vi "Update VI Properties.vi"() -> ()   [LabVIEW 2016, in "update vi properties.lvlib"]
uses:
  update vi properties.lvlib
  support/user action.ctl
  support/Event Data.ctl
  support/Cluster_Data.ctl
  <vilib>/picture/picture.llb/imagedata.ctl
panel:
  in  "Adjust all Controls & Indicators":bool=TRUE
  in  "Prompt?":bool
  in  "Set all VIs":bool
  in  "Load":bool
  in  "Error in":errorcluster
  in  "Event Data":T1
  in  "Controls":string[][](table)
  in  "Indicators":string[][](table)
  in  "Help Tag":string
  in  "Help Path":string
  out "Path to VI":string
  in  "VI Description":string
  out "VI Conn Pane":picture
  in  "Select a VI to View/Edit Properties:":i32(listbox)=-1
  in  "Action":T2
  in  "OK":bool
  in  "Cancel":bool
  in  "Apply":bool
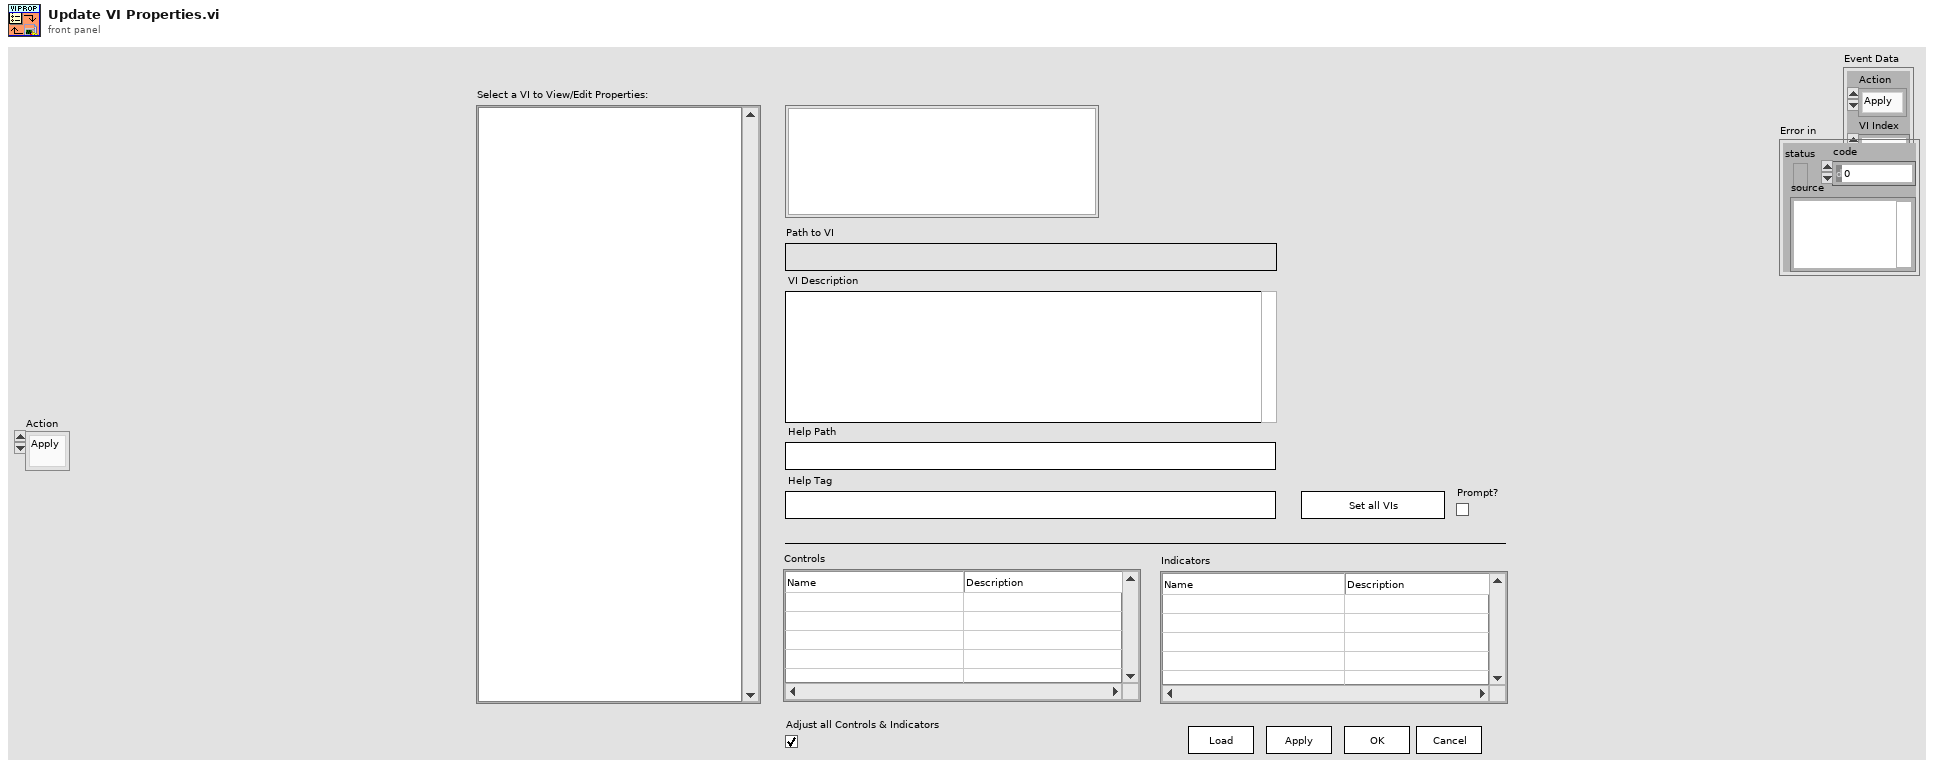
[diagram p1: front panel]
types:
  T1 = typedef "update vi properties.lvlib/Event Data.ctl" = cluster{"Action":T2, "VI Index":i32}
  T2 = typedef "update vi properties.lvlib/user action.ctl" = enum16{"Apply", "Cancel", "VI Selected", "Value Changed", "Set all VIs", "Controls/Indicator Changed", "Load VIs"}
  T3 = typedef "update vi properties.lvlib/Cluster_Data.ctl" = cluster{"changed?":bool, "VI Data":string[], "Controls":string[][], "Indicator":string[][], "Conpane Img":T4}
  T4 = typedef "imagedata.ctl" = cluster{"image type":i32, "image depth":i32, "image":u8[], "mask":u8[], "colors":u32[], "Rectangle":cluster{"left":i16, "top":i16, "right":i16, "bottom":i16}}
  T5 = enum32{"invalid VI type", "Standard VI", "Control VI", "Global VI", "Polymorphic VI", "Configuration VI", "SubSystem", "Facade VI", "Method VI", "Statechart Diagram VI"}
  T6 = enum8{"Enabled", "Disabled", "Disabled and Grayed Out"}
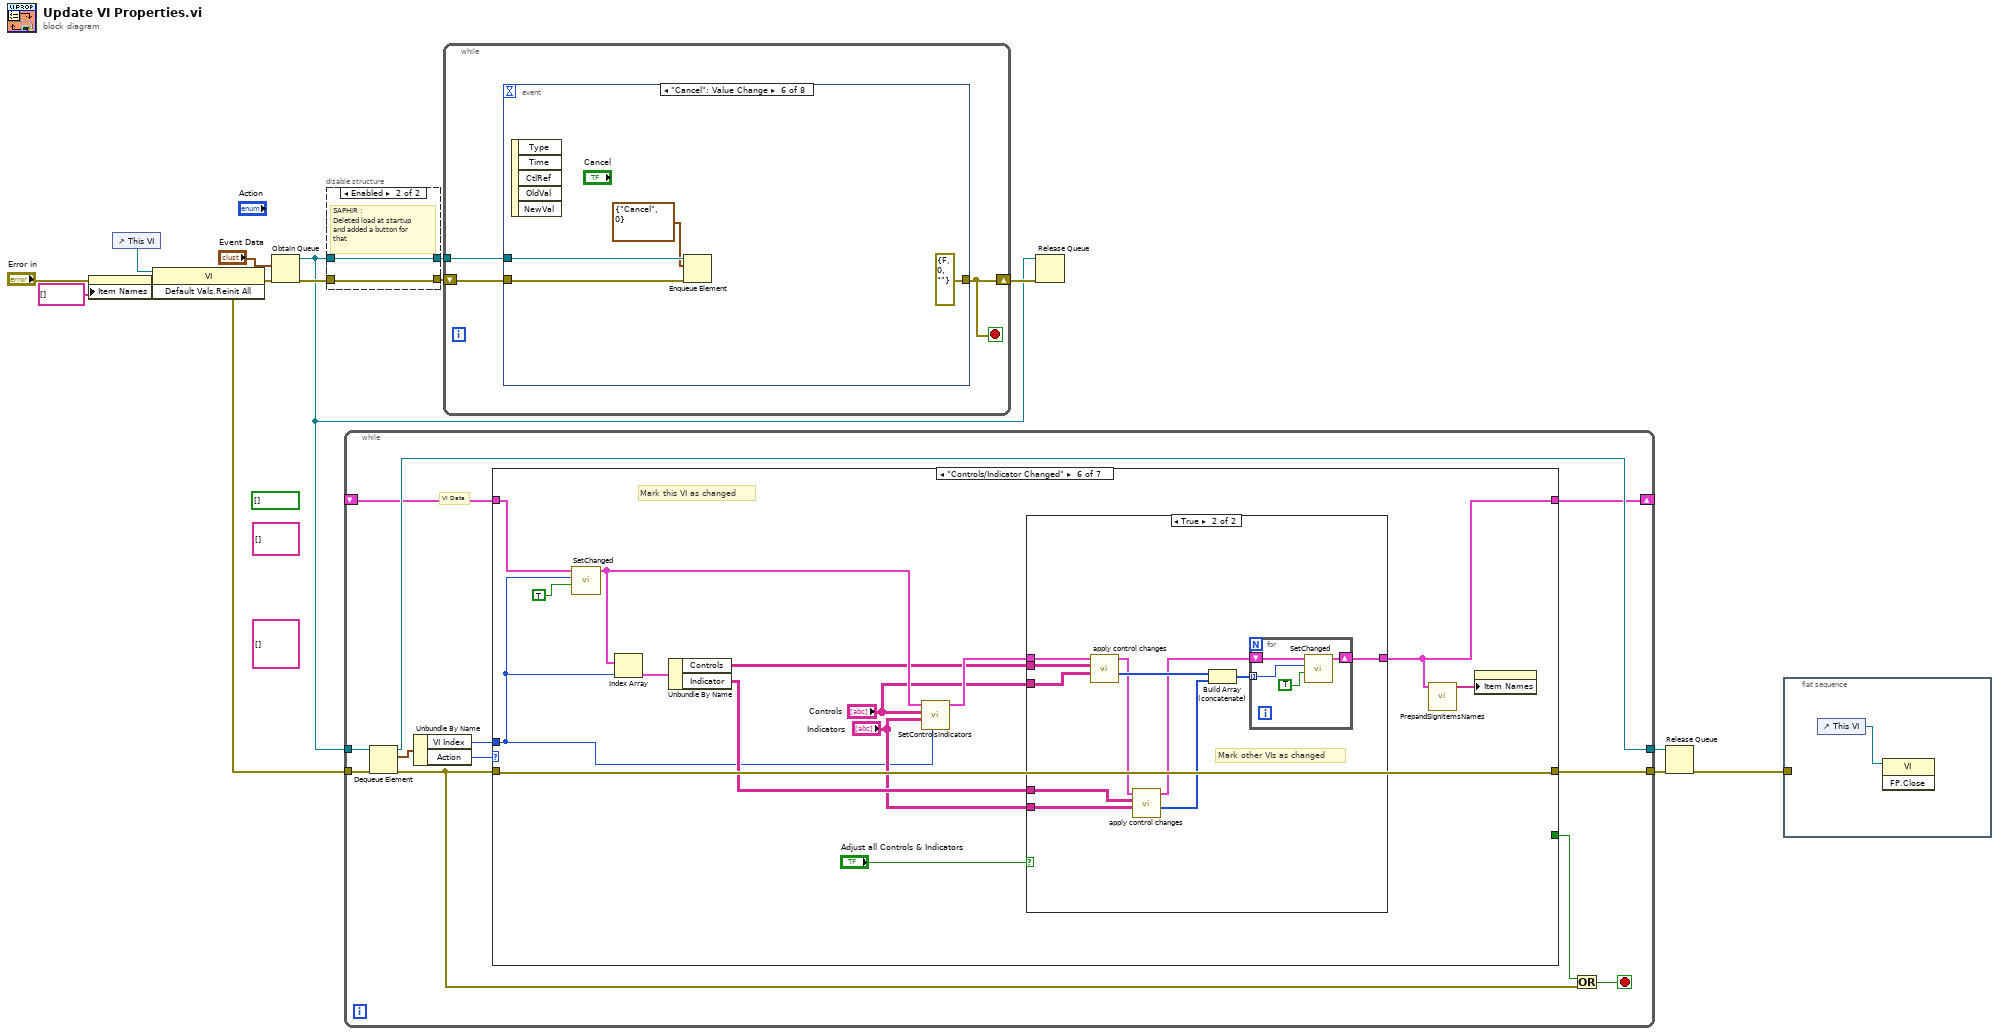
[diagram p0: block diagram]
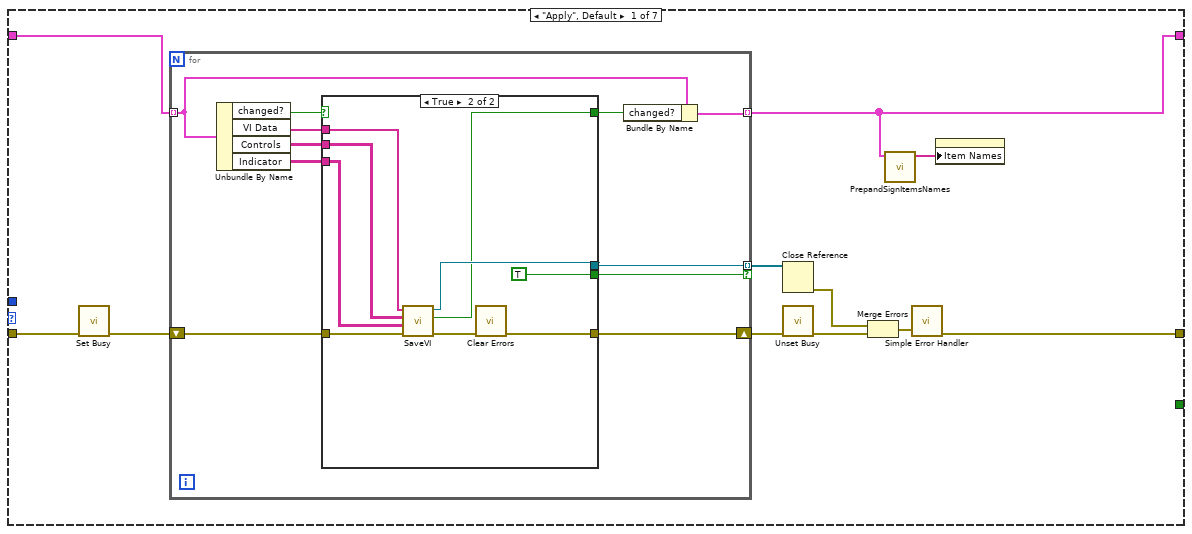
[diagram p2: hidden frame]
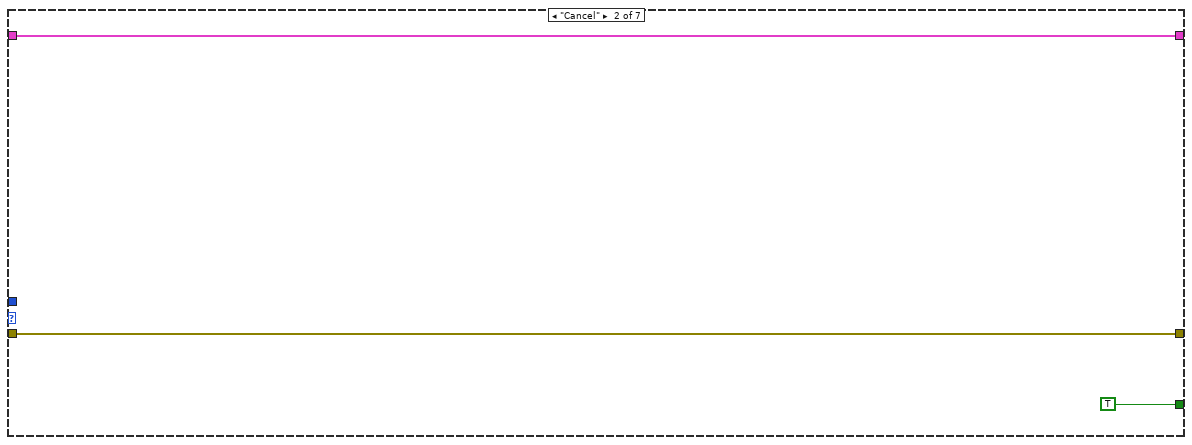
[diagram p4: hidden frame]
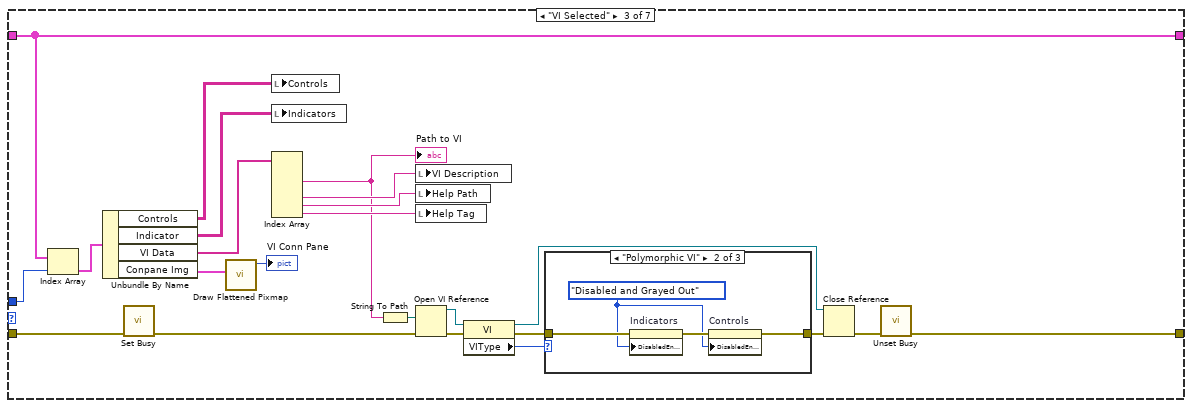
[diagram p5: hidden frame]
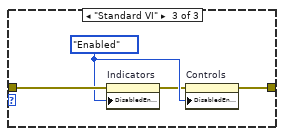
[diagram p7: hidden frame]
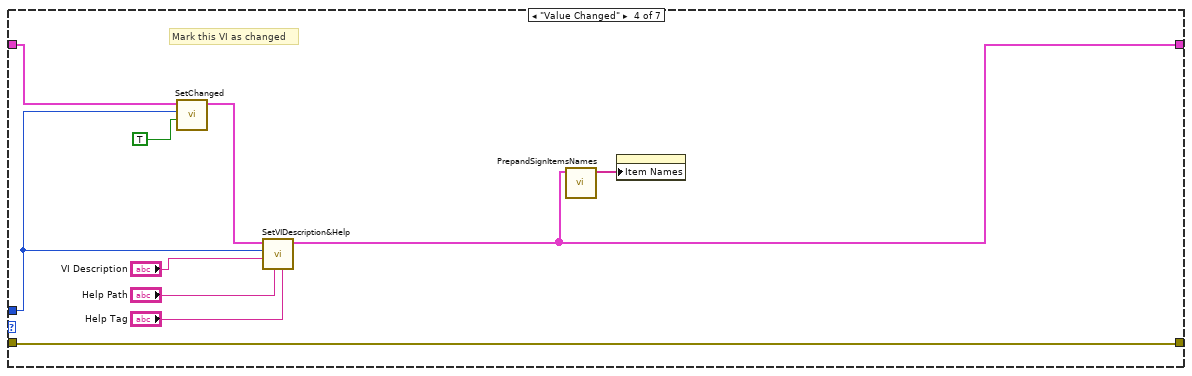
[diagram p8: hidden frame]
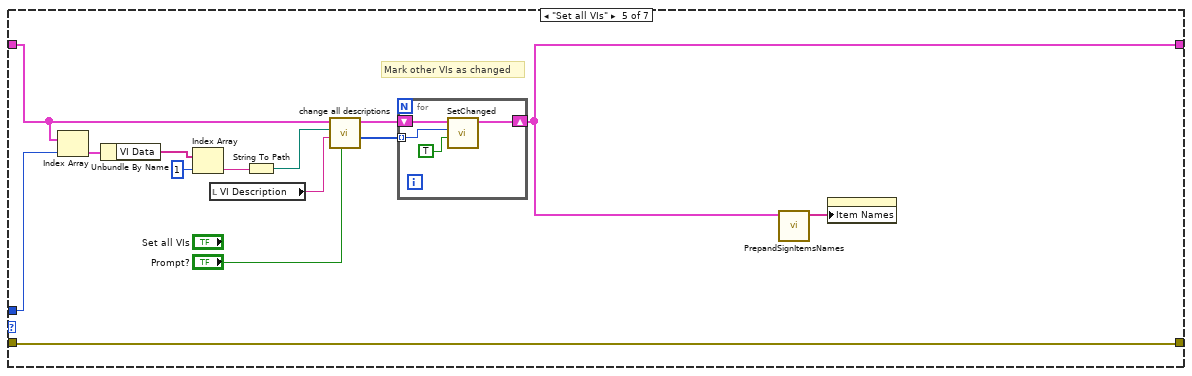
[diagram p9: hidden frame]
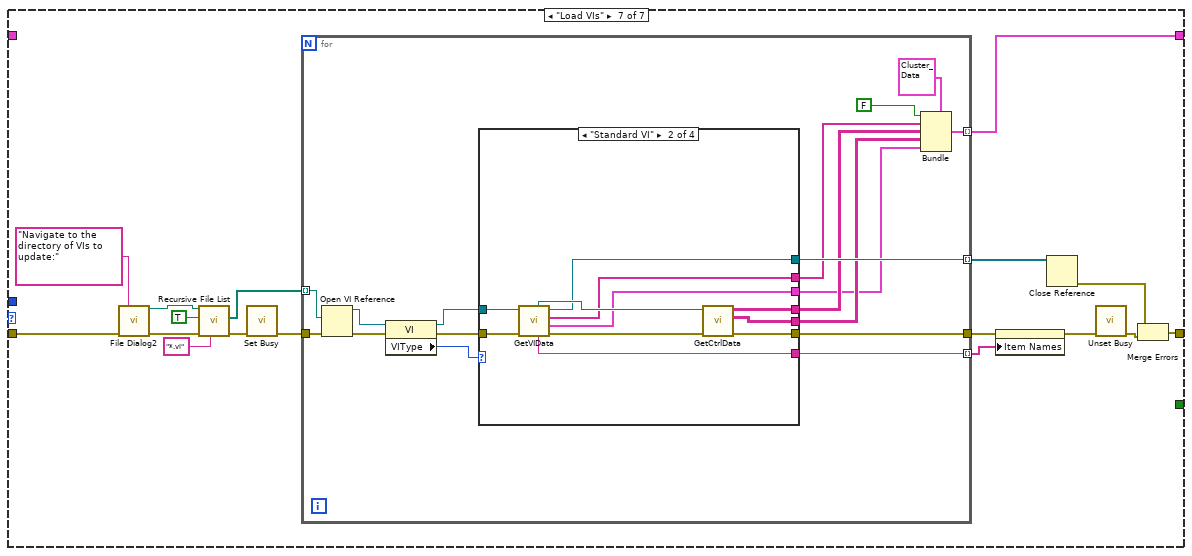
[diagram p11: hidden frame]
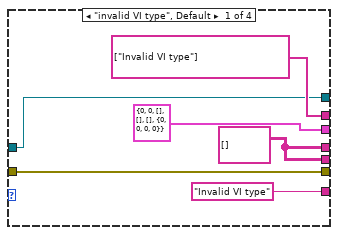
[diagram p12: hidden frame]
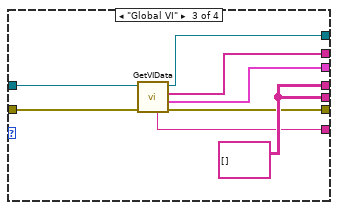
[diagram p13: hidden frame]
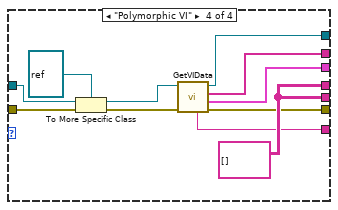
[diagram p14: hidden frame]
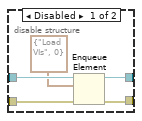
[diagram p15: hidden frame]
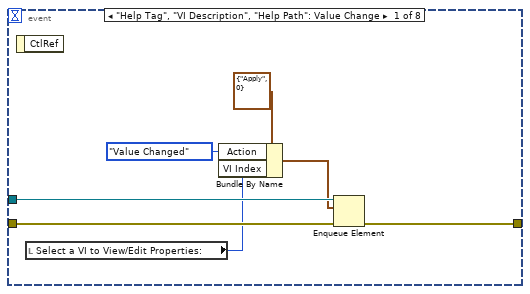
[diagram p16: hidden frame]
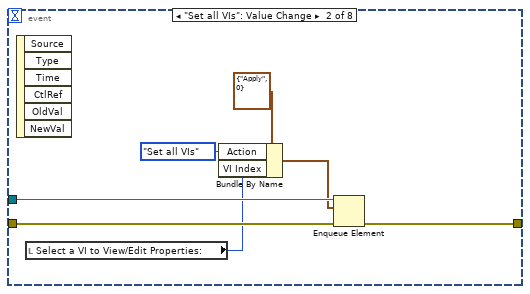
[diagram p17: hidden frame]
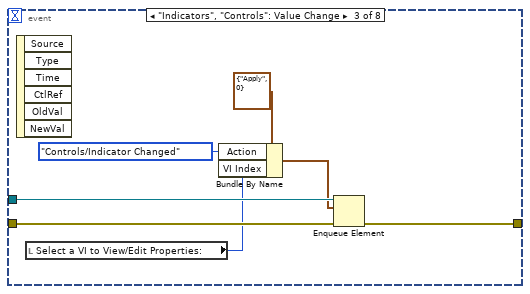
[diagram p18: hidden frame]
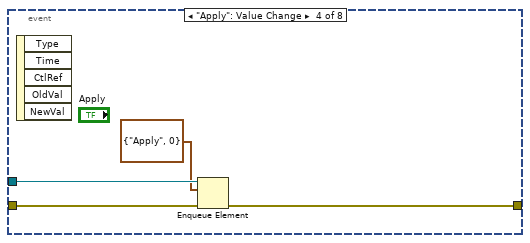
[diagram p19: hidden frame]
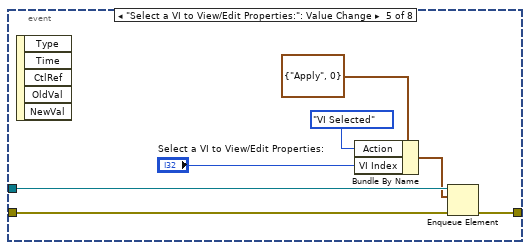
[diagram p20: hidden frame]
diagram:
  (unwired) string[][][] []
  (unwired) string[][] []
  (unwired) bool[] []
  n1 = property on="Select a VI to View/Edit Properties:" class="LstBox (strict)"(error in="Error in", "Item Names"=string[] []) -> (error out=w5:errorcluster)  [unwired: 1 in, 1 out]
  n2 = control-ref of="This VI"() -> (w8:refnum<vi>)
  n3 = invoke class="VI" method="Default Vals.Reinit All"(reference=w8, error in=w5) -> (error out=w7:errorcluster)  [unwired: 1 in, 2 out]
  n4 = Obtain Queue(element data type="Event Data", error in (no error)=w7) -> (queue out=w2:refnum<queue>, error out=w11:errorcluster)  [unwired: 3 in, 1 out]
  n5 = disable-structure shown="Enabled" {
    disable-tunnel: w11 -> [w19 w21]
    disable-tunnel: [w18 w21] -> w10
    disable-tunnel: w2 -> [w17 w20]
    disable-tunnel: [w16 w20] -> w9
    frame Disabled {
      n6 = Enqueue Element(queue=w17, element=T1 {"Action"=enum."Load VIs", "VI Index"=0}, error in (no error)=w19) -> (queue out=w16:refnum<queue>, error out=w18:errorcluster)  [unwired: 1 in, 1 out]
    }
    frame Enabled {
      # "SAPHIR :\nDeleted load at startup\nand added a button for\nthat"
    }
  }
  n7 = while {
    tunnel: w7 -> [w29]
    tunnel: w2 -> [w33]
    tunnel: [w26] -> w14
    tunnel: [w32] -> w13
    shift-right: [w27] -> _
    shift-left: _ -> [w28]
    stop <- w23 stop-if-true
    # "VI Data"
    n8 = Dequeue Element(queue=w33, error in (no error)=w29) -> (queue out=w32:refnum<queue>, element=w31:T1, error out=w24:errorcluster)  [unwired: 1 in, 1 out]
    n9 = Unbundle By Name(w31) -> ("VI Index"=w30:i32, "Action"=w25:T2)
    n10 = case shown="\"Controls/Indicator Changed\"" w25 {
      tunnel: w24 -> [w44 w70 w89 w113 w127 w145 w174]
      tunnel: [_ TRUE _ _ _ _ _] -> w22
      tunnel: [w37 w70 w77 w113 w127 w145 w163] -> w26
      tunnel: w30 -> [_ _ w88 w110 w116 w134 _]
      tunnel: w28 -> [w36 w69 w76 w108 w124 w141 _]
      tunnel: [w34 w69 w76 w104 w115 w132 w162] -> w27
      frame "Apply", Default {
        n11 = call <vilib>:"Set Busy.vi"("error in (no error)"=w44) -> ("error out"=w43:errorcluster)  [unwired: 9 in, 1 out]
        n12 = for {
          shift-right: [w53] -> w42
          shift-left: w43 -> [w55]
          tunnel: w36 -> [w50] mode=indexing
          tunnel: [w54] -> w40 mode=indexing if=w52
          tunnel: [w48] -> w34 mode=indexing
          n13 = Unbundle By Name(w50) -> ("changed?"=w51:bool, "VI Data"=w47:string[], "Controls"=w46:string[][], "Indicator"=w45:string[][])
          n14 = case shown="True" w51 {
            selector: w51 -> [w56 _]
            tunnel: w47 -> [_ w68]
            tunnel: w55 -> [w58 w67]
            tunnel: [refnum<k0> refnum w66] -> w54
            tunnel: [w58 w65] -> w53
            tunnel: [FALSE TRUE] -> w52
            tunnel: [w56 w62] -> w49
            tunnel: w46 -> [_ w61]
            tunnel: w45 -> [_ w60]
            frame False {
            }
            frame True {
              n15 = call "SaveVI.vi"("error in (no error)"=w67, "Indicator"=w60, "Controls"=w61, "Data"=w68) -> ("error out"=w63:errorcluster, "status"=w62:bool, "VI out"=w66:refnum<vi>)  [unwired: 5 in]
              n16 = call <vilib>:"Clear Errors.vi"("error in (no error)"=w63) -> ("error out"=w65:errorcluster)  [unwired: 5 in, 1 out]
            }
          }
          n17 = Bundle By Name(cluster=w50, "changed?"=w49) -> (w48:T3)
        }
        n18 = Close Reference(reference=w40) -> (error out=w38:errorcluster)  [unwired: 1 in]
        n19 = call <vilib>:"Unset Busy.vi"("error in (no error)"=w42) -> ("error out"=w41:errorcluster)  [unwired: 10 in]
        n20 = Merge Errors(w38, w41) -> (w39:errorcluster)
        n21 = call "PrepandSignItemsNames.vi"("VI Data in"=w34) -> ("Array"=w35:string[])  [unwired: 10 in]
        n22 = call <vilib>:"Simple Error Handler.vi"("error in (no error)"=w39) -> ("error out"=w37:errorcluster)  [unwired: 4 in, 4 out]
        n23 = property on="Select a VI to View/Edit Properties:" class="LstBox (strict)"("Item Names"=w35) -> ()  [unwired: 2 in, 2 out]
      }
      frame "Cancel" {
      }
      frame "VI Selected" {
        n24 = Index Array(array=w76, index=w88) -> (element=w93:T3)
        n25 = Unbundle By Name(w93) -> ("Controls"=w72:string[][], "Indicator"=w73:string[][], "VI Data"=w74:string[], "Conpane Img"=w75:T4)
        n26 = call <vilib>:"Set Busy.vi"("error in (no error)"=w89) -> ("error out"=w78:errorcluster)  [unwired: 9 in, 1 out]
        n27 = call <vilib>:"Draw Flattened Pixmap.vi"("image data"=w75) -> ("new picture"=→"VI Conn Pane":picture)  [unwired: 8 in]
        n28 = local write "Controls"(w72) -> ()
        n29 = local write "Indicators"(w73) -> ()
        n30 = Index Array(array=w74) -> (element #2=w87:string, element #4=w92:string, element #5=w91:string, element #6=w90:string)  [unwired: 6 in, 2 out]
        "Path to VI" <- w87
        n31 = String To Path(string=w87) -> (path=w86:path)
        n32 = local write "VI Description"(w92) -> ()
        n33 = local write "Help Path"(w91) -> ()
        n34 = local write "Help Tag"(w90) -> ()
        n35 = Open VI Reference(vi path=w86, error in (no error)=w78) -> (vi reference=w85:refnum<vi>, error out=w84:errorcluster)  [unwired: 4 in]
        n36 = property class="VI"(reference=w85, error in=w84) -> (reference out=w79:refnum<vi>, error out=w82:errorcluster, "VIType"=w83:T5)
        n37 = case shown="\"Polymorphic VI\"" w83 {
          tunnel: w82 -> [w95 w98 w103]
          tunnel: [w95 w97 w100] -> w81
          frame "invalid VI type", Default {
          }
          frame "Polymorphic VI" {
            w96 = T6."Disabled and Grayed Out" ("Disabled")
            n38 = property on="Indicators" class="Tbl (strict)"(error in=w98, "DisabledEnum"=w96) -> (error out=w99:errorcluster)  [unwired: 1 in, 1 out]
            n39 = property on="Controls" class="Tbl (strict)"(error in=w99, "DisabledEnum"=w96) -> (error out=w97:errorcluster)  [unwired: 1 in, 1 out]
          }
          frame "Standard VI" {
            w102 = T6."Enabled" ("Disabled")
            n40 = property on="Indicators" class="Tbl (strict)"(error in=w103, "DisabledEnum"=w102) -> (error out=w101:errorcluster)  [unwired: 1 in, 1 out]
            n41 = property on="Controls" class="Tbl (strict)"(error in=w101, "DisabledEnum"=w102) -> (error out=w100:errorcluster)  [unwired: 1 in, 1 out]
          }
        }
        n42 = Close Reference(reference=w79, error in (no error)=w81) -> (error out=w80:errorcluster)
        n43 = call <vilib>:"Unset Busy.vi"("error in (no error)"=w80) -> ("error out"=w77:errorcluster)  [unwired: 10 in]
      }
      frame "Value Changed" {
        # "Mark this VI as changed"
        n44 = call "SetChanged.vi"("changed?"=TRUE ("new element/subarray"), "VI Index"=w110, "Array in"=w108) -> ("Array out"=w107:T3[])  [unwired: 8 in]
        n45 = call "SetVIDescription&Help.vi"("Help Tag"="Help Tag", "Help Path"="Help Path", "VI Description"="VI Description", "VI Index"=w110, "VI Data in"=w107) -> ("VI Data out"=w104:T3[])  [unwired: 6 in]
        n46 = call "PrepandSignItemsNames.vi"("VI Data in"=w104) -> ("Array"=w105:string[])  [unwired: 10 in]
        n47 = property on="Select a VI to View/Edit Properties:" class="LstBox (strict)"("Item Names"=w105) -> ()  [unwired: 2 in, 2 out]
      }
      frame "Set all VIs" {
        # "Mark other VIs as changed"
        n48 = Index Array(array=w124, index=w116) -> (element=w123:T3)
        n49 = Unbundle By Name(w123) -> ("VI Data"=w122:string[])
        n50 = Index Array(array=w122, index=1) -> (element=w120:string)
        n51 = local read "VI Description"() -> (w118:string)
        n52 = String To Path(string=w120) -> (path=w119:path)
        n53 = call "change all descriptions.vi"("Prompt?"="Prompt?", "new"=w118, "Path"=w119, "VI Data in"=w124) -> ("Changed indices"=w126:i32[], "VI Data out"=w125:T3[])  [unwired: 5 in, 1 out]
        n54 = for {
          shift-right: [w130] -> w115
          shift-left: w125 -> [w131]
          tunnel: w126 -> [w129] mode=indexing
          n55 = call "SetChanged.vi"("changed?"=TRUE ("new element/subarray"), "VI Index"=w129, "Array in"=w131) -> ("Array out"=w130:T3[])  [unwired: 8 in]
        }
        n56 = call "PrepandSignItemsNames.vi"("VI Data in"=w115) -> ("Array"=w114:string[])  [unwired: 10 in]
        n57 = property on="Select a VI to View/Edit Properties:" class="LstBox (strict)"("Item Names"=w114) -> ()  [unwired: 2 in, 2 out]
      }
      frame "Controls/Indicator Changed" {
        # "Mark this VI as changed"
        n58 = call "SetChanged.vi"("changed?"=TRUE ("new element/subarray"), "VI Index"=w134, "Array in"=w141) -> ("Array out"=w138:T3[])  [unwired: 8 in]
        n59 = Index Array(array=w138, index=w134) -> (element=w144:T3)
        n60 = Unbundle By Name(w144) -> ("Controls"=w137:string[][], "Indicator"=w139:string[][])
        n61 = call "SetControlsIndicators.vi"("VI Index"=w134, "Indicators"="Indicators", "Controls"="Controls", "Data In"=w138) -> ("Data Out"=w143:T3[])  [unwired: 7 in]
        n62 = case shown="True" "Adjust all Controls & Indicators" {
          tunnel: "Controls" -> [_ w156]
          tunnel: w137 -> [_ w157]
          tunnel: w139 -> [_ w155]
          tunnel: "Indicators" -> [_ w154]
          tunnel: w143 -> [w146 w149]
          tunnel: [w146 w151] -> w132
          frame False {
          }
          frame True {
            # "Mark other VIs as changed"
            n63 = call "apply control changes.vi"("new"=w156, "old"=w157, "Data In"=w149) -> ("Changed indices"=w153:i32[], "Data Out"=w148:T3[])  [unwired: 7 in]
            n64 = call "apply control changes.vi"("new"=w154, "old"=w155, "Data In"=w148) -> ("Changed indices"=w152:i32[], "Data Out"=w147:T3[])  [unwired: 7 in]
            n65 = Build Array (concatenate)(w153, w152) -> (w150:i32[])
            n66 = for {
              shift-right: [w160] -> w151
              shift-left: w147 -> [w161]
              tunnel: w150 -> [w159] mode=indexing
              n67 = call "SetChanged.vi"("changed?"=TRUE ("new element/subarray"), "VI Index"=w159, "Array in"=w161) -> ("Array out"=w160:T3[])  [unwired: 8 in]
            }
          }
        }
        n68 = call "PrepandSignItemsNames.vi"("VI Data in"=w132) -> ("Array"=w133:string[])  [unwired: 10 in]
        n69 = property on="Select a VI to View/Edit Properties:" class="LstBox (strict)"("Item Names"=w133) -> ()  [unwired: 2 in, 2 out]
      }
      frame "Load VIs" {
        n70 = call "File Dialog2"("prompt"="Navigate to the directory of VIs to update:", "error in"=w174) -> ("selected path"=w176:path, "error out"=w177:errorcluster)  [unwired: 10 in, 2 out]
        n71 = call <vilib>:"Recursive File List.vi"("pattern"="*.vi", "error in (no error)"=w177, "Treat LLBs as Folders?"=TRUE, "Folder Path"=w176) -> ("error out"=w172:errorcluster, "All Files in Dir"=w170:path[])  [unwired: 3 in, 3 out]
        n72 = call <vilib>:"Set Busy.vi"("error in (no error)"=w172) -> ("error out"=w171:errorcluster)  [unwired: 9 in, 1 out]
        n73 = for {
          tunnel: w171 -> [w193]
          tunnel: w170 -> [w192] mode=indexing
          tunnel: [w188] -> w169 mode=indexing
          tunnel: [w187] -> w168
          tunnel: [w186] -> w166 mode=indexing
          tunnel: [w180] -> w162 mode=indexing
          n74 = Open VI Reference(vi path=w192, error in (no error)=w193) -> (vi reference=w195:refnum<vi>, error out=w194:errorcluster)  [unwired: 4 in]
          n75 = property class="VI"(reference=w195, error in=w194) -> (reference out=w190:refnum<vi>, error out=w191:errorcluster, "VIType"=w189:T5)
          n76 = case shown="\"Standard VI\"" w189 {
            tunnel: w191 -> [w197 w212 w220 w230]
            tunnel: w190 -> [w196 w211 w214 w229]
            tunnel: [string[] ["Invalid VI type"] w202 w216 w223] -> w185
            tunnel: ["Invalid VI type" ("Name") w204 w217 w225] -> w188
            tunnel: [w199 w207 w219 w228] -> w184
            tunnel: [w199 w206 w219 w228] -> w183
            tunnel: [T4 {"image type"=0, "image depth"=0, "image"=[], "mask"=[], "colors"=[], "Rectangle"={"left"=0, "top"=0, "right"=0, "bottom"=0}} ("Get Conpane Image") w205 w215 w222] -> w182
            tunnel: [w197 w203 w218 w224] -> w187
            tunnel: [w196 w208 w213 w221] -> w186
            frame "invalid VI type", Default {
              w199 = string[][] []
            }
            frame "Standard VI" {
              n77 = call "GetVIData.vi"("error in (no error)"=w212, "VI in"=w211) -> ("error out"=w210:errorcluster, "Get Conpane Image"=w205:T4, "Array"=w202:string[], "VI out"=w208:refnum<vi>, "Name"=w204:string, "Panel"=w209:refnum<vi>)  [unwired: 4 in]
              n78 = call "GetCtrlData.vi"("error in (no error)"=w210, "Panel in"=w209) -> ("error out"=w203:errorcluster, "Indicators"=w206:string[][], "Controls"=w207:string[][])  [unwired: 7 in]
            }
            frame "Global VI" {
              w219 = string[][] []
              n79 = call "GetVIData.vi"("error in (no error)"=w220, "VI in"=w214) -> ("error out"=w218:errorcluster, "Get Conpane Image"=w215:T4, "Array"=w216:string[], "VI out"=w213:refnum<vi>, "Name"=w217:string)  [unwired: 4 in, 1 out]
            }
            frame "Polymorphic VI" {
              w228 = string[][] []
              n80 = To More Specific Class(target class=refnum<vi> refnum, reference=w229, error in=w230) -> (specific class reference=w226:refnum<vi>, error out=w227:errorcluster)
              n81 = call "GetVIData.vi"("error in (no error)"=w227, "VI in"=w226) -> ("error out"=w224:errorcluster, "Get Conpane Image"=w222:T4, "Array"=w223:string[], "VI out"=w221:refnum<vi>, "Name"=w225:string)  [unwired: 4 in, 1 out]
            }
          }
          n82 = Bundle(cluster=T3 {"changed?"=FALSE, "VI Data"=[], "Controls"=[], "Indicator"=[], "Conpane Img"={"image type"=0, "image depth"=0, "image"=[], "mask"=[], "colors"=[], "Rectangle"={"left"=0, "top"=0, "right"=0, "bottom"=0}}}, "changed?"=FALSE, "VI Data"=w185, "Controls"=w184, "Indicator"=w183, "Conpane Img"=w182) -> (w180:T3)
        }
        n83 = property on="Select a VI to View/Edit Properties:" class="LstBox (strict)"(error in=w168, "Item Names"=w169) -> (error out=w167:errorcluster)  [unwired: 1 in, 1 out]
        n84 = Close Reference(reference=w166) -> (error out=w165:errorcluster)  [unwired: 1 in]
        n85 = call <vilib>:"Unset Busy.vi"("error in (no error)"=w167) -> ("error out"=w164:errorcluster)  [unwired: 10 in]
        n86 = Merge Errors(w165, w164) -> (w163:errorcluster)
      }
    }
    n87 = Or(x=w22, y=w24) -> (x .or. y?=w23:bool)
  }
  n88 = while {
    shift-right: [w232] -> w3
    shift-left: w10 -> [w233]
    tunnel: w9 -> [w234]
    stop <- w232 stop-if-true
    n89 = event shown="[5] \"Cancel\": Value Change" {
      selector: _ -> [_ _ _ _ _ _ _ _]
      dyn-events: _ -> [_ _ _ _ _ _ _ _]
      timeout: _ -> [_ _ _ _ _ _ _ _]
      tunnel: w234 -> [w241 w248 w255 w259 w266 w270 w276 w280]
      tunnel: w233 -> [w240 w247 w254 w258 w265 w269 w277 w279]
      tunnel: [w239 w246 w253 w257 w261 errorcluster {"status"=FALSE, "code"=0, "source"=""} ("error out") w273 w278] -> w232
      event "Help Tag", "VI Description", "Help Path": Value Change {
        n90 = event-data() -> ()  [unwired: 1 in, 1 out]
        n91 = local read "Select a VI to View/Edit Properties:"() -> (w236:i32)
        n92 = Bundle By Name(cluster=T1 {"Action"=enum."Apply", "VI Index"=0} ("element"), "Action"=user_action."Value Changed", "VI Index"=w236) -> (w235:T1)
        n93 = Enqueue Element(queue=w241, element=w235, error in (no error)=w240) -> (error out=w239:errorcluster)  [unwired: 1 in, 2 out]
      }
      event "Set all VIs": Value Change {
        n94 = event-data() -> ()  [unwired: 1 in, 6 out]
        n95 = local read "Select a VI to View/Edit Properties:"() -> (w243:i32)
        n96 = Bundle By Name(cluster=T1 {"Action"=enum."Apply", "VI Index"=0} ("element"), "Action"=user_action."Set all VIs", "VI Index"=w243) -> (w242:T1)
        n97 = Enqueue Element(queue=w248, element=w242, error in (no error)=w247) -> (error out=w246:errorcluster)  [unwired: 1 in, 2 out]
      }
      event "Indicators", "Controls": Value Change {
        n98 = event-data() -> ()  [unwired: 1 in, 6 out]
        n99 = local read "Select a VI to View/Edit Properties:"() -> (w250:i32)
        n100 = Bundle By Name(cluster=T1 {"Action"=enum."Apply", "VI Index"=0} ("element"), "Action"=user_action."Controls/Indicator Changed", "VI Index"=w250) -> (w249:T1)
        n101 = Enqueue Element(queue=w255, element=w249, error in (no error)=w254) -> (error out=w253:errorcluster)  [unwired: 1 in, 2 out]
      }
      event "Apply": Value Change {
        n102 = event-data() -> ()  [unwired: 1 in, 5 out]
        n103 = Enqueue Element(queue=w259, element=T1 {"Action"=enum."Apply", "VI Index"=0}, error in (no error)=w258) -> (error out=w257:errorcluster)  [unwired: 1 in, 2 out]
      }
      event "Select a VI to View/Edit Properties:": Value Change {
        n104 = event-data() -> ()  [unwired: 1 in, 5 out]
        n105 = Bundle By Name(cluster=T1 {"Action"=enum."Apply", "VI Index"=0} ("element"), "Action"=user_action."VI Selected", "VI Index"="Select a VI to View/Edit Properties:") -> (w262:T1)
        n106 = Enqueue Element(queue=w266, element=w262, error in (no error)=w265) -> (error out=w261:errorcluster)  [unwired: 1 in, 2 out]
      }
      event "Cancel": Value Change {
        n107 = event-data() -> ()  [unwired: 1 in, 5 out]
        n108 = Enqueue Element(queue=w270, element=T1 {"Action"=enum."Cancel", "VI Index"=0}, error in (no error)=w269) -> ()  [unwired: 1 in, 3 out]
      }
      event "OK": Value Change {
        (unwired) FALSE ("Cancel")
        n109 = event-data() -> ()  [unwired: 1 in, 5 out]
        n110 = Enqueue Element(queue=w276, element=T1 {"Action"=enum."Apply", "VI Index"=0}, error in (no error)=w277) -> (queue out=w274:refnum<queue>, error out=w275:errorcluster)  [unwired: 1 in, 1 out]
        n111 = Enqueue Element(queue=w274, element=T1 {"Action"=enum."Cancel", "VI Index"=0}, error in (no error)=w275) -> (error out=w273:errorcluster)  [unwired: 1 in, 2 out]
      }
      event "Load": Value Change {
        n112 = event-data() -> ()  [unwired: 1 in, 5 out]
        n113 = Enqueue Element(queue=w280, element=T1 {"Action"=enum."Load VIs", "VI Index"=0}, error in (no error)=w279) -> (error out=w278:errorcluster)  [unwired: 1 in, 2 out]
      }
    }
  }
  n114 = Release Queue(queue=w2, error in (no error)=w3) -> ()  [unwired: 1 in, 3 out]
  n115 = Release Queue(queue=w13, error in (no error)=w14) -> (error out=w1:errorcluster)  [unwired: 1 in, 2 out]
  n116 = flat-sequence {
    tunnel: w1 -> [_]
    frame #0 {
      n117 = control-ref of="This VI"() -> (w282:refnum<vi>)
      n118 = invoke class="VI" method="FP.Close"(reference=w282) -> ()  [unwired: 2 in, 3 out]
    }
  }
